vi "Request Data JSON.vi"(8 "error in (no error)":errorcluster, 11 "CallVendorRequest in":refnum<class "CallVendorRequest.lvclass">) -> (0 "error out":errorcluster, 2 "Request Data JSON":string, 3 "CallVendorRequest out":refnum<class "CallVendorRequest.lvclass">)   [LabVIEW 2022 SP3, in "obs-websocket-lv.lvlib" / "CallVendorRequest.lvclass"]
uses:
  CallVendorRequest.lvclass
  CallVendorRequest.lvclass/CallVendorRequest.ctl
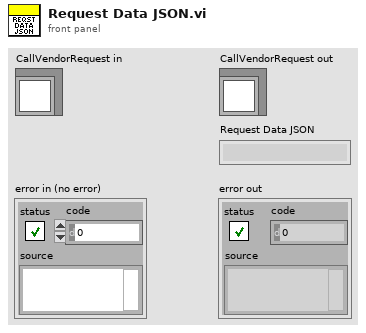
[diagram p1: front panel]
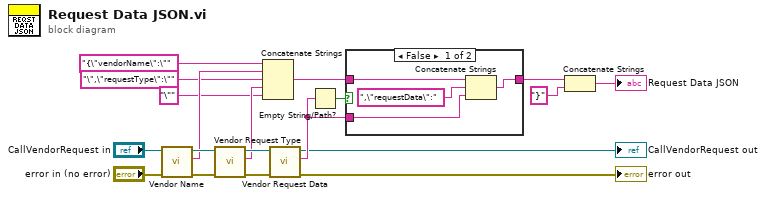
[diagram p0: block diagram]
diagram:
  n1 = call-dynamic "Vendor Name.vi"("error in (no error)"="error in (no error)", "CallVendorRequest in"="CallVendorRequest in") -> ("error out"=w16:errorcluster, "Vendor Name"=w12:string, "CallVendorRequest out"=w17:refnum<class "CallVendorRequest.lvclass">)  [unwired: 7 in]
  n2 = call-dynamic "Vendor Request Type.vi"("error in (no error)"=w16, "CallVendorRequest in"=w17) -> ("error out"=w14:errorcluster, "Vendor Request Type"=w10:string, "CallVendorRequest out"=w15:refnum<class "CallVendorRequest.lvclass">)  [unwired: 7 in]
  n3 = Concatenate Strings("{\"vendorName\":\"" ("string"), w12, "\",\"requestType\":\"" ("string"), w10, "\"" ("string")) -> (w8:string)
  n4 = call-dynamic "Vendor Request Data.vi"("error in (no error)"=w14, "CallVendorRequest in"=w15) -> ("error out"=→"error out":errorcluster, "Vendor Request Data JSON"=w6:string, "CallVendorRequest out"=→"CallVendorRequest out":refnum<class "CallVendorRequest.lvclass">)  [unwired: 7 in]
  n5 = Empty String/Path?(string/path=w6) -> (empty?=w7:bool)
  n6 = case shown="False" w7 {
    tunnel: w8 -> [w23 w24]
    tunnel: w6 -> [w21 _]
    tunnel: [w20 w24] -> w5
    frame False {
      n7 = Concatenate Strings(w23, ",\"requestData\":" ("string"), w21) -> (w20:string)
    }
    frame True {
    }
  }
  n8 = Concatenate Strings(w5, "}" ("string")) -> (→"Request Data JSON":string)
